vi "InitAll1.vi"() -> ()   [LabVIEW 2018]
panel:
  in  "停止":bool
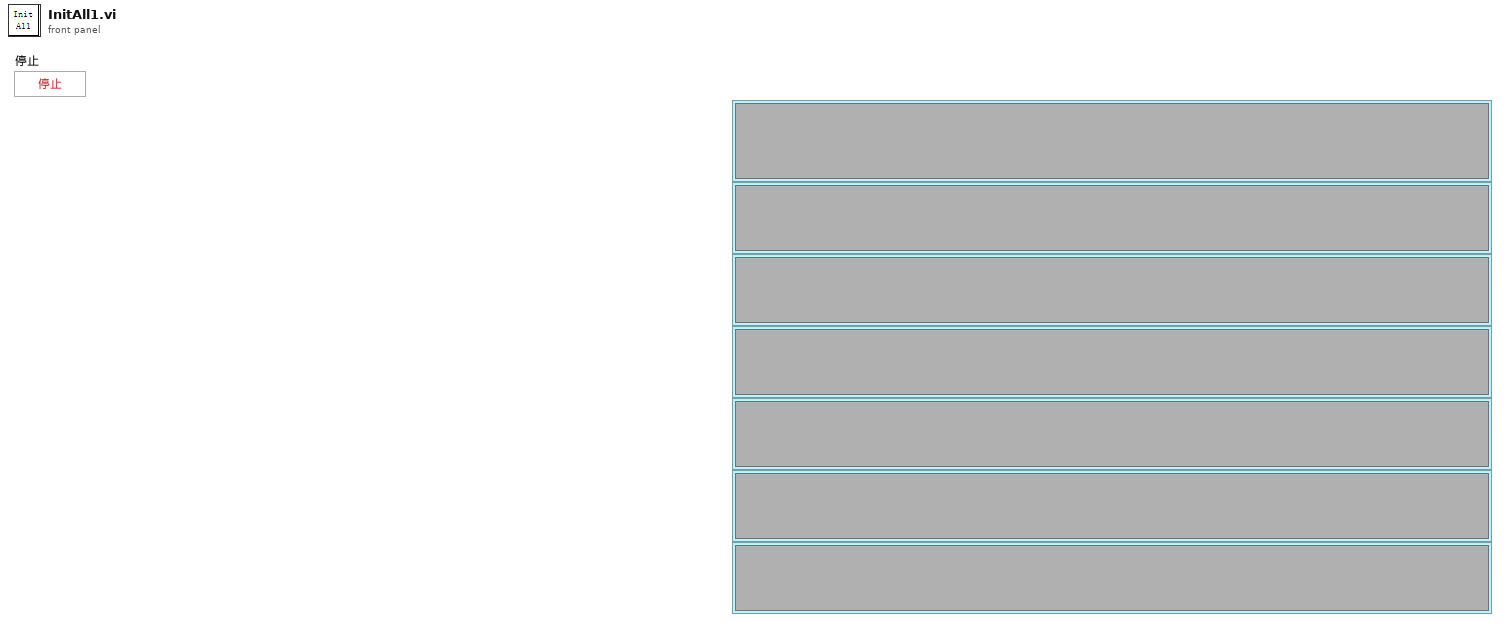
[diagram p1: front panel]
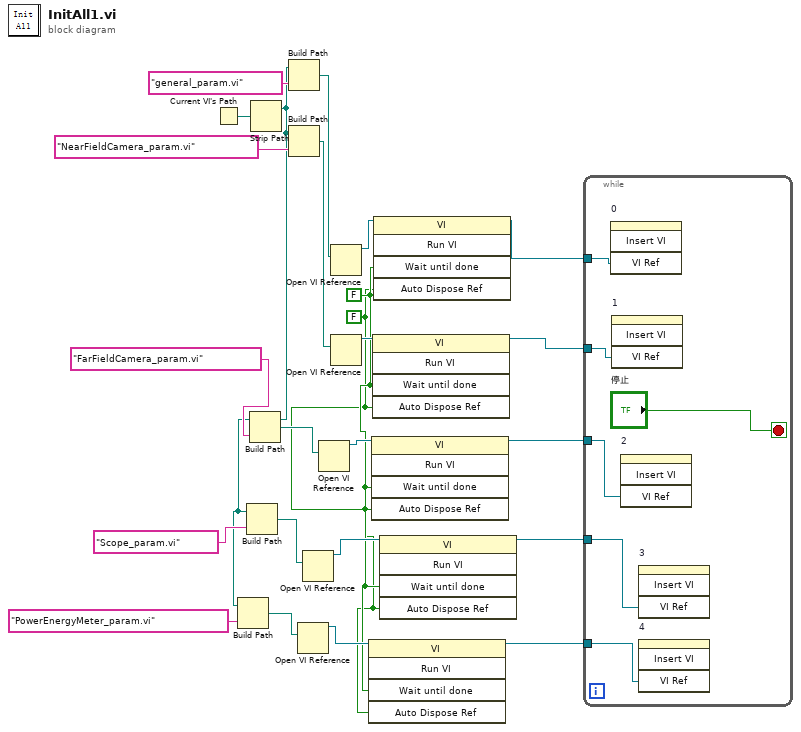
[diagram p0: block diagram]
diagram:
  w2 = FALSE ("自动销毁引用")
  w3 = FALSE ("结束前等待")
  n1 = Current VI's Path() -> (path=w22:path)
  n2 = Strip Path(path=w22) -> (stripped path=w7:path)  [unwired: 1 out]
  n3 = Build Path(base path=w7, name or relative path="PowerEnergyMeter_param.vi" ("名称或相对路径")) -> (appended path=w5:path)
  n4 = Build Path(base path=w7, name or relative path="Scope_param.vi" ("名称或相对路径")) -> (appended path=w9:path)
  n5 = Build Path(base path=w7, name or relative path="FarFieldCamera_param.vi" ("名称或相对路径")) -> (appended path=w14:path)
  n6 = Build Path(base path=w7, name or relative path="general_param.vi" ("名称或相对路径")) -> (appended path=w19:path)
  n7 = Build Path(base path=w7, name or relative path="NearFieldCamera_param.vi" ("名称或相对路径")) -> (appended path=w18:path)
  n8 = Open VI Reference(vi path=w5) -> (vi reference=w4:refnum<vi>)  [unwired: 5 in, 1 out]
  n9 = Open VI Reference(vi path=w9) -> (vi reference=w10:refnum<vi>)  [unwired: 5 in, 1 out]
  n10 = Open VI Reference(vi path=w14) -> (vi reference=w15:refnum<vi>)  [unwired: 5 in, 1 out]
  n11 = Open VI Reference(vi path=w19) -> (vi reference=w24:refnum<vi>)  [unwired: 5 in, 1 out]
  n12 = Open VI Reference(vi path=w18) -> (vi reference=w17:refnum<vi>)  [unwired: 5 in, 1 out]
  n13 = invoke class="VI" method="Run VI"(reference=w4, "Wait until done"=w3, "Auto Dispose Ref"=w2) -> (reference out=w1:refnum<vi>)  [unwired: 2 in, 4 out]
  n14 = invoke class="VI" method="Run VI"(reference=w15, "Wait until done"=w3, "Auto Dispose Ref"=w2) -> (reference out=w12:refnum<vi>)  [unwired: 2 in, 4 out]
  n15 = invoke class="VI" method="Run VI"(reference=w17, "Wait until done"=w3, "Auto Dispose Ref"=w2) -> (reference out=w16:refnum<vi>)  [unwired: 2 in, 4 out]
  n16 = invoke class="VI" method="Run VI"(reference=w24, "Wait until done"=w3, "Auto Dispose Ref"=w2) -> (reference out=w23:refnum<vi>)  [unwired: 2 in, 4 out]
  n17 = invoke class="VI" method="Run VI"(reference=w10, "Wait until done"=w3, "Auto Dispose Ref"=w2) -> (reference out=w8:refnum<vi>)  [unwired: 2 in, 4 out]
  n18 = while {
    tunnel: w23 -> [w29]
    tunnel: w16 -> [w28]
    tunnel: w12 -> [w27]
    tunnel: w8 -> [w26]
    tunnel: w1 -> [w25]
    stop <- "停止" stop-if-true
    n19 = invoke on="0" class="SubPnl" method="Insert VI"("VI Ref"=w29) -> ()  [unwired: 3 in, 4 out]
    n20 = invoke on="1" class="SubPnl" method="Insert VI"("VI Ref"=w28) -> ()  [unwired: 3 in, 4 out]
    n21 = invoke on="2" class="SubPnl" method="Insert VI"("VI Ref"=w27) -> ()  [unwired: 3 in, 4 out]
    n22 = invoke on="3" class="SubPnl" method="Insert VI"("VI Ref"=w26) -> ()  [unwired: 3 in, 4 out]
    n23 = invoke on="4" class="SubPnl" method="Insert VI"("VI Ref"=w25) -> ()  [unwired: 3 in, 4 out]
  }
